vi "Load Plugin Prepare.vi"(6 "Version String":string, 8 "error in (no error)":errorcluster, 9 "Unique Name":string, 10 "Plugin Type":string="CIFTemplatePlugin", 11 "Launcher in":refnum<class "CIFPluginManager.lvclass">) -> (0 "error out":errorcluster, 1 "Unique Name (dup)":string, 2 "Matching Plugin":T1, 3 "Launcher (dup)":refnum<class "CIFPluginManager.lvclass">, 5 "path":path)   [LabVIEW 2021, in "CIFPluginManager.lvclass"]
doc: "This prepares the loading action. Because the VI server process can be slow it is moved outside of the Load Plugin Prepare process to the Load Plugin Action. The prepare will detect most common configuration errors. This allows the UI to get any configuration errors returned but not need to wait for the full load to complete."
uses:
  CIFPluginManager.lvclass
  CIFCore/Common/Typedef/Errors.ctl
  CIFPluginManager.lvclass/CIFPluginManager.ctl
  CIFUtilities/CIFConfigurationFile/typedef/Location Type.ctl
  <vilib>/CIF Foundation/CIF Utilities/Errors/Append Error Location.vi
  CIFUtilities/CIFConfigurationFile/CIF Configuration File Location.vi
  <vilib>/CIF Foundation/CIF Utilities/Time/System Time/LabVIEW Time to TAI Time.vi
  <vilib>/Utility/LVLibp/NI_PackedLibraryUtility.lvlib
  CIFCore/Common/CIFCoreCommon.lvlib
  CIFUtilities/CIFConfigurationFile/CIF Configuration File.lvlib
  CIFCore/Common/Typedef/Version.ctl
  typedef/Plugin Metadata.ctl
  typedef/Discovered Plugin.ctl
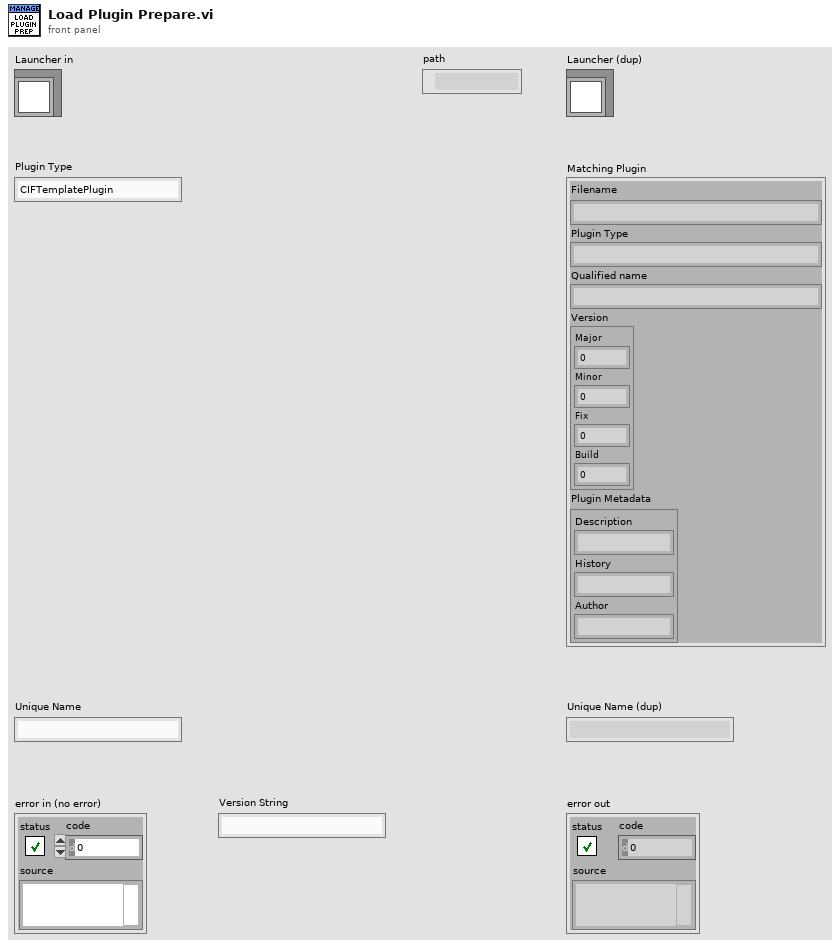
[diagram p1: front panel]
types:
  T1 = typedef "CIFPluginManager.lvclass/Discovered Plugin.ctl" = cluster{"Filename":string, "Plugin Type":string, "Qualified name":string, "Version":T2, "Plugin Metadata":T3}
  T2 = typedef "CIFCoreCommon.lvlib/Version.ctl" = cluster{"Major":i32, "Minor":i32, "Fix":i32, "Build":i32}
  T3 = typedef "CIFPluginManager.lvclass/Plugin Metadata.ctl" = cluster{"Description":string, "History":string, "Author":string}
  T4 = typedef "CIFCoreCommon.lvlib/Errors.ctl" = enum16{"Invalid Clock ID", "Long Sleep", "gRPC Server Not Found", "Config Parse", "Timestamp Wrap", "Delayed Execution", "Duplicate Channel", "Missing Channel", "Incorrect Type", "Flatten Error", "Unflatten Data", "Unique Name", "Plugin Not Found", "Plugin Type Not Found", "Plugin Version Not Found", "Manager Not Found", "Numerical Issue", "Time Jump", "Clock ID Match", "Channel Length", "Plugin Connection", "gRPC Server Connection", "PPL Name Match", "Build", "Config Log Parse", "Plugin Load", "UI Subpanel Load", "Python Name", "Invalid Name", "Unable to Change Ch Buffer"}
  T5 = typedef "CIF Configuration File.lvlib/Location Type.ctl" = enum16{"Config File", "Manager", "Protos", "Plugins", "UI Plugins", "Logs", "Orchestrations"}
  T6 = typedef "CIFPluginManager.lvclass/Plugin Management Data.ctl" = cluster{"vi reference":refnum<vi>, "gRPC ID":T7, "Plugin Type":string, "Unique Name":string, "gRPC Port":i32, "Version":T2, "Load Timestamp":i64, "Unload Timestamp":i64, "Unloading":bool, "Ready for removal":bool, "status":T8}
  T7 = typedef "grpc-lvsupport-release.lvlib/grpcId.ctl" = u64
  T8 = typedef "CIF_Manager_server.lvlib/cif_plugincore_StatusData.ctl" = cluster{"state":T9, "timing_statistics":T10, "fifo_statistics":T12, "error":T13, "monitor_doubles":T14, "monitor_u64s":T15, "monitor_i64s":T16}
  T9 = typedef "CIF_Manager_server.lvlib/cif_plugincore_StatusData_State.ctl" = enum32{"NULL", "CREATING", "LISTENING", "RUNNING", "CLEANINGUP", "DESTROYING"}
  T10 = typedef "CIF_Manager_server.lvlib/cif_plugincore_TimingStatistics.ctl" = cluster{"period":T11, "wake_error":T11, "execute":T11, "housekeep":T11, "idle":T11, "cleanup":T11, "custom_1":T11, "custom_2":T11}
  T11 = typedef "CIF_Manager_server.lvlib/cif_common_TimingStats.ctl" = cluster{"max":i64, "min":i64, "avg":dbl}
  T12 = typedef "CIF_Manager_server.lvlib/cif_plugincore_FifoStatistics.ctl" = cluster{"from_t0":T11, "from_previous_plugin":T11, "output_error":T11}
  T13 = typedef "CIF_Manager_server.lvlib/cif_plugincore_Error.ctl" = cluster{"status":bool, "code":i32}
  T14 = typedef "CIF_Manager_server.lvlib/cif_plugincore_MonitorDoubles.ctl" = cluster{"double_1":dbl, "double_2":dbl, "double_3":dbl, "double_4":dbl}
  T15 = typedef "CIF_Manager_server.lvlib/cif_plugincore_MonitorU64.ctl" = cluster{"u64_1":u64, "u64_2":u64, "u64_3":u64, "u64_4":u64}
  T16 = typedef "CIF_Manager_server.lvlib/cif_plugincore_MonitorI64.ctl" = cluster{"i64_1":i64, "i64_2":i64, "i64_3":i64, "i64_4":i64}
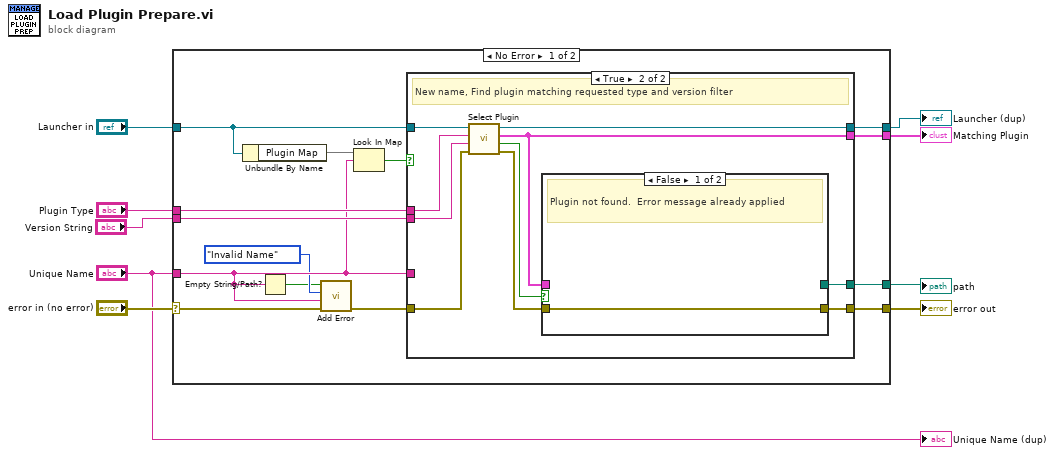
[diagram p0: block diagram]
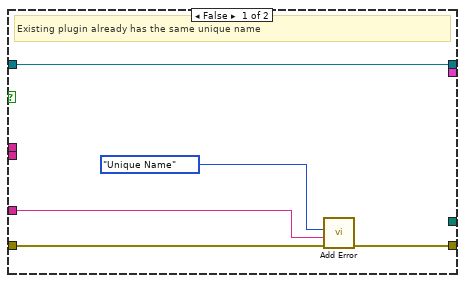
[diagram p2: hidden frame]
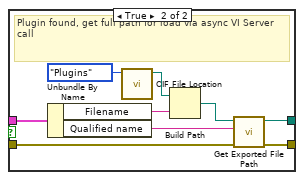
[diagram p3: hidden frame]
diagram:
  n1 = case shown="No Error" "error in (no error)" {
    selector: "error in (no error)" -> [w17 w50]
    tunnel: [w23 w50] -> w8
    tunnel: "Launcher in" -> [w18 w49]
    tunnel: "Plugin Type" -> [w22 _]
    tunnel: "Unique Name" -> [w15 _]
    tunnel: "Version String" -> [w19 _]
    tunnel: [w12 _] -> w3
    tunnel: [w11 _] -> w2
    tunnel: [w10 w49] -> w1
    frame No Error {
      n2 = Unbundle By Name(w18) -> ("Plugin Map"=w21:map{string, T6})
      n3 = Empty String/Path?(string/path=w15) -> (empty?=w13:bool)
      n4 = call "Add Error.vi"("error in (no error)"=w17, "String to Append"=w15, "Error"=Errors."Invalid Name", "Insert Error"=w13) -> ("error out"=w16:errorcluster)  [unwired: 7 in]
      n5 = Look In Map(map=w21, key=w15) -> (key not found?=w20:bool)  [unwired: 1 in, 1 out]
      n6 = case shown="True" w20 {
        tunnel: w16 -> [w28 w34]
        tunnel: [w25 w38] -> w23
        tunnel: w22 -> [_ w36]
        tunnel: w15 -> [w26 _]
        tunnel: w18 -> [w24 w37]
        tunnel: w19 -> [_ w35]
        tunnel: [_ w30] -> w12
        tunnel: [_ w31] -> w11
        tunnel: [w24 w29] -> w10
        frame False {
          # "Existing plugin already has the same unique name"
          n7 = call "Add Error.vi"("error in (no error)"=w28, "String to Append"=w26, "Error"=Errors."Unique Name") -> ("error out"=w25:errorcluster)  [unwired: 8 in]
        }
        frame True {
          # "New name, Find plugin matching requested type and version filter"
          n8 = call "Select Plugin.vi"("error in (no error)"=w34, "Version String"=w35, "Plugin Type"=w36, "CIFPluginManager in"=w37) -> ("error out"=w33:errorcluster, "Match found"=w32:bool, "Matching Plugin"=w30:T1, "CIFPluginManager out"=w29:refnum<class "CIFPluginManager.lvclass">)  [unwired: 4 in]
          n9 = case shown="False" w32 {
            tunnel: [w39 w42] -> w38
            tunnel: w33 -> [w39 w47]
            tunnel: w30 -> [_ w41]
            tunnel: [_ w40] -> w31
            frame False {
              # "Plugin not found.  Error message already applied"
            }
            frame True {
              # "Plugin found, get full path for load via async VI Server call"
              n10 = Unbundle By Name(w41) -> ("Filename"=w46:string, "Qualified name"=w45:string)
              n11 = call "CIF File Location.vi"("LocationType"=Location_Type."Plugins") -> ("Location"=w43:path)  [unwired: 10 in]
              n12 = Build Path(base path=w43, name or relative path=w46) -> (appended path=w48:path)
              n13 = call <vilib>:"Get Exported File Path.vi"("error in (no error)"=w47, "qualified name"=w45, "packed library path"=w48) -> ("error out"=w42:errorcluster, "path"=w40:path)  [unwired: 7 in]
            }
          }
        }
      }
    }
    frame Error {
    }
  }
  "error out" <- w8
  "Matching Plugin" <- w3
  "path" <- w2
  "Launcher (dup)" <- w1
  "Unique Name (dup)" <- "Unique Name"
